vi "alignRight.vi"(6 "ignoreCaption&Labels":bool, 8 "error in (no error)":errorcluster, 11 "refs":refnum<vi>[](array[refnum])) -> (0 "error out":errorcluster, 3 "refs(dup)":refnum<vi>[](array[refnum]))   [LabVIEW 2023, in "TLC_Geometry.lvlib"]
doc: "Aligns all controls to the topmost position among the input controls.\nThe topmost coordinate is computed and applied to all controls."
uses:
  TLC_Geometry.lvlib
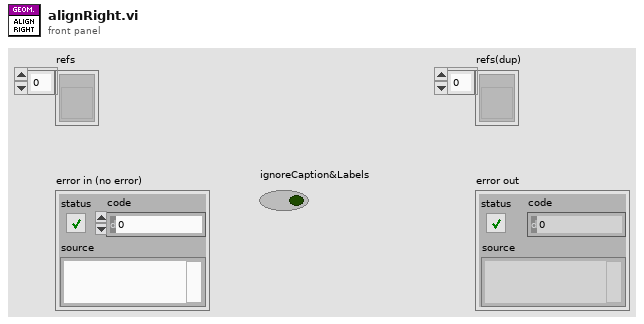
[diagram p1: front panel]
types:
  T1 = cluster{"left":i32, "top":i32, "right":i32, "bottom":i32}
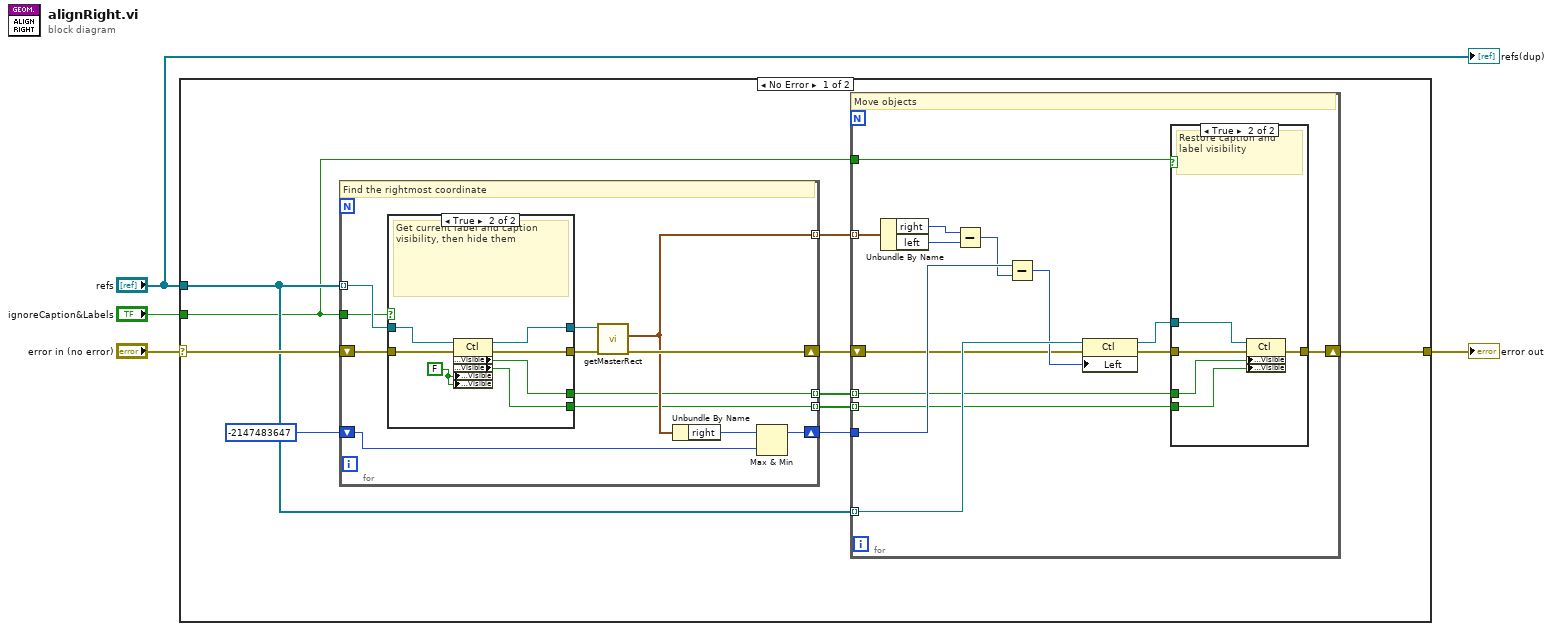
[diagram p0: block diagram]
diagram:
  n1 = case shown="No Error" "error in (no error)" {
    selector: "error in (no error)" -> [w14 w56]
    tunnel: [w11 w56] -> w3
    tunnel: "refs" -> [w12 _]
    tunnel: "ignoreCaption&Labels" -> [w7 _]
    frame No Error {
      n2 = for {
        tunnel: w12 -> [w40] mode=indexing
        shift-right: [w46] -> w10
        shift-left: w14 -> [w39]
        shift-right: [w43] -> w9
        shift-left: -2147483647 -> [w44]
        tunnel: [w42] -> w8 mode=indexing
        tunnel: w7 -> [w37]
        tunnel: [w36] -> w6 mode=indexing
        tunnel: [w35] -> w5 mode=indexing
        # "Find the rightmost coordinate"
        n3 = case shown="True" w37 {
          tunnel: [w48 w55] -> w41
          tunnel: w40 -> [w48 w54]
          tunnel: w39 -> [w47 w53]
          tunnel: [w47 w52] -> w38
          tunnel: [_ w51] -> w36
          tunnel: [_ w50] -> w35
          frame False {
            # "Do nothing"
          }
          frame True {
            w49 = FALSE ("Caption.Visible")
            # "Get current label and caption visibility, then hide them"
            n4 = property class="Ctl"(reference=w54, error in=w53, "Caption.Visible"=w49, "Label.Visible"=w49) -> (reference out=w55:refnum<vi>, error out=w52:errorcluster, "Caption.Visible"=w51:bool, "Label.Visible"=w50:bool)
          }
        }
        n5 = call "getMasterRect.vi"("error in (no error)"=w38, "ref"=w41) -> ("error out"=w46:errorcluster, "rect"=w42:T1)  [unwired: 7 in, 1 out]
        n6 = Unbundle By Name(w42) -> ("right"=w45:i32)
        n7 = Max & Min(x=w45, y=w44) -> (max(x,y)=w43:i32)  [unwired: 1 out]
      }
      n8 = for {
        tunnel: w12 -> [w28] mode=indexing
        shift-right: [w20] -> w11
        shift-left: w10 -> [w21]
        tunnel: w9 -> [w24]
        tunnel: w8 -> [w27] mode=indexing
        tunnel: w7 -> [w18]
        tunnel: w6 -> [w16] mode=indexing
        tunnel: w5 -> [w15] mode=indexing
        # "Move objects"
        n9 = Unbundle By Name(w27) -> ("right"=w26:i32, "left"=w25:i32)
        n10 = Subtract(x=w26, y=w25) -> (x-y=w23:i32)
        n11 = Subtract(x=w24, y=w23) -> (x-y=w22:i32)
        n12 = property class="Ctl"(reference=w28, error in=w21, "Left"=w22) -> (reference out=w17:refnum<vi>, error out=w19:errorcluster)
        n13 = case shown="True" w18 {
          tunnel: w17 -> [_ w34]
          tunnel: w19 -> [w29 w33]
          tunnel: [w29 w32] -> w20
          tunnel: w16 -> [_ w31]
          tunnel: w15 -> [_ w30]
          frame False {
            # "Do nothing"
          }
          frame True {
            # "Restore caption and label visibility"
            n14 = property class="Ctl"(reference=w34, error in=w33, "Caption.Visible"=w31, "Label.Visible"=w30) -> (error out=w32:errorcluster)  [unwired: 1 out]
          }
        }
      }
    }
    frame Error {
    }
  }
  "error out" <- w3
  "refs(dup)" <- "refs"
